vi "addData.vi"(8 "error in (no error)":errorcluster, 10 "Data":u8[](array[numeric]), 11 "DynamicFrameBuilder in":refnum<class "DynamicFrameBuilder.lvclass">) -> (0 "error out":errorcluster, 3 "DynamicFrameBuilder out":refnum<class "DynamicFrameBuilder.lvclass">)   [LabVIEW 2016, in "RTModbus.lvlib" / "DynamicFrameBuilder.lvclass"]
uses:
  DynamicFrameBuilder.lvclass
  DynamicFrameBuilder.lvclass/DynamicFrameBuilder.ctl
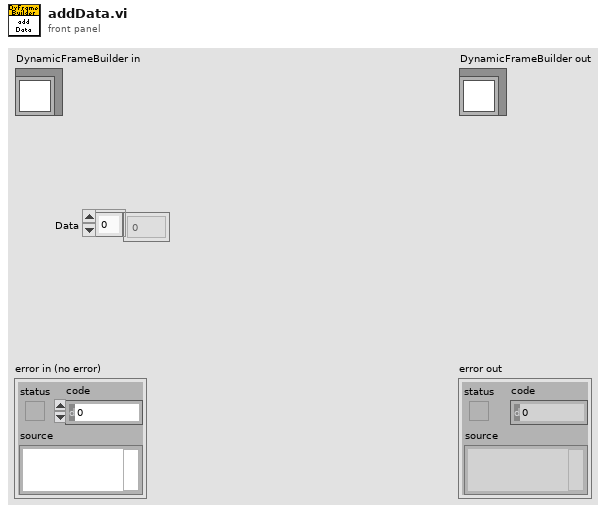
[diagram p1: front panel]
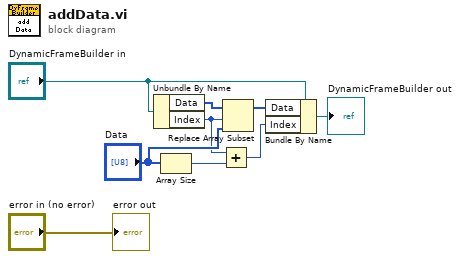
[diagram p0: block diagram]
diagram:
  n1 = Unbundle By Name("DynamicFrameBuilder in") -> ("Data"=w6:u8[], "Index"=w1:i32)
  n2 = Array Size(array="Data") -> (size(s)=w3:i32)
  n3 = Add(x=w1, y=w3) -> (x+y=w2:i32)
  n4 = Replace Array Subset(array=w6, new element="Data", index=w1) -> (w5:u8[])
  n5 = Bundle By Name(cluster="DynamicFrameBuilder in", "Data"=w5, "Index"=w2) -> (→"DynamicFrameBuilder out":refnum<class "DynamicFrameBuilder.lvclass">)
  "error out" <- "error in (no error)"
